vi "Wait till chilled water below.vi"(3 "Mode":T5, 5 "Traverse line In":T2 {"Carrier_2 Q (l/min)" format="%#.2f"; "Row Duration (mins)" format="%#.1f"; "Row No" min=0; "Trace Gas Concentration (%)" min=0.0 format="%#_4f"; "Carrier_1 Q (l/min)" format="%#.4f"; "Tunnel Speed" format="%#.2f"; "Start X" format="%#.2f"; "Start Y" format="%#.2f"; "Start Z" format="%#.2f"; "End X" format="%#.2f"; "End Y" format="%#.2f"; "End Z" format="%#.2f"; "Averaging time (min)" min=0.0 format="%#.2f"}) -> (0 "Error Message":string, 1 "Status":T1, 2 "Traverse line Out":T2 {"Carrier_2 Q (l/min)" format="%#.2f"; "Row Duration (mins)" format="%#.1f"; "Row No" min=0; "Trace Gas Concentration (%)" min=0.0 format="%#_4f"; "Carrier_1 Q (l/min)" format="%#.4f"; "Tunnel Speed" format="%#.2f"; "Start X" format="%#.2f"; "Start Y" format="%#.2f"; "Start Z" format="%#.2f"; "End X" format="%#.2f"; "End Y" format="%#.2f"; "End Z" format="%#.2f"; "Averaging time (min)" min=0.0 format="%#.2f"})   [LabVIEW 2020]
uses:
  Gen Trav/Multi_Run_Status.ctl
  Controls/User_Specific_mode.ctl
  ADAM Client/Sub VIs/ADAM Controls/Tunnel_speed_mode.ctl
  Gen Trav/Spacing.ctl
  Gen Trav/Traverse_cluster.ctl
  Controls/Multi_run_mode.ctl
panel:
  out "Initial Hydrosonic setting":dbl
  in  "stop":bool
  out "Chilled water temp":dbl(graph)
  out "Initial Uni Chilled water temp":dbl
  out "Initial Tunnel Speed":dbl
  # "X           Y            Z"
  # "Start"
  # "End"
  # "X           Y            Z"
  # "Start"
  # "End"
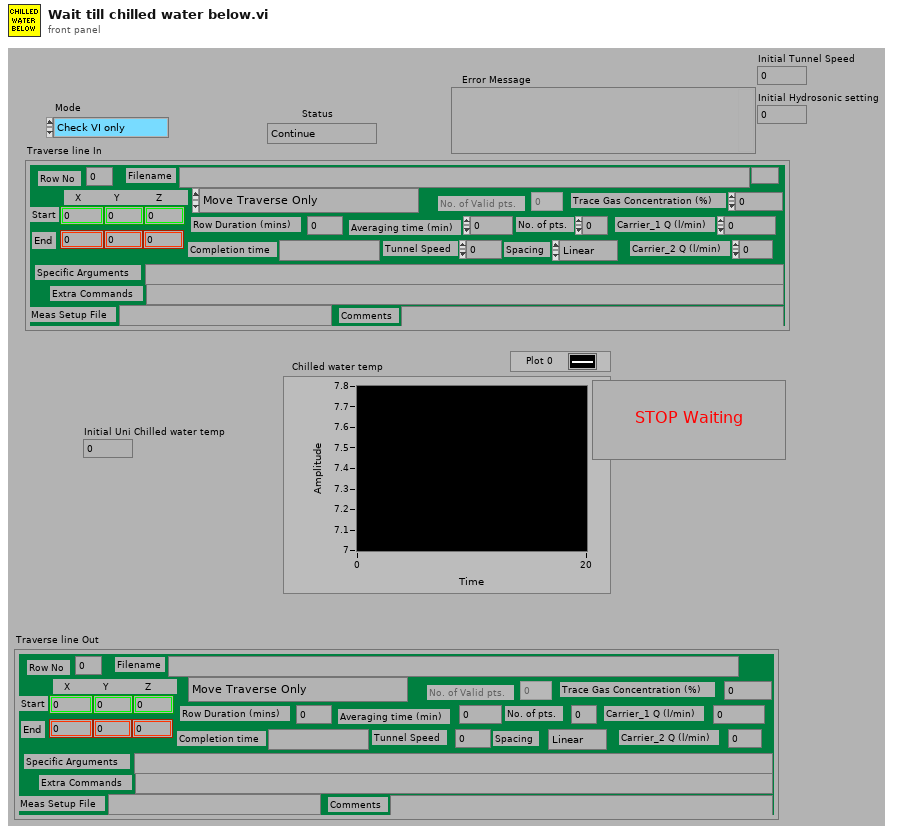
[diagram p1: front panel]
types:
  T1 = typedef "Multi_Run_Status.ctl" = enum16{"Continue", "Continue with Error", "Jump to Next Point", "Jump to Next Row", "Jump To Fall Back", "Terminate Run"}
  T2 = typedef "Traverse_cluster.ctl" = cluster{"Start X":sgl, "Start Y":sgl, "Start Z":sgl, "End X":sgl, "End Y":sgl, "End Z":sgl, "No. of pts.":i32, "Spacing":T3, "Filename":path, "Tunnel Speed":dbl, "Averaging time (min)":dbl, "Extra Commands":string, "Carrier_1 Q (l/min)":dbl, "Carrier_2 Q (l/min)":dbl, "Trace Gas Concentration (%)":dbl, "Specific Arguments":string, "Comments":string, "Row No":i32, "Row Type Selector":T4, "Completion time":string, "Row Duration (mins)":dbl, "No. of Valid pts.":i32, "Meas Setup File":string}
  T3 = typedef "Spacing.ctl" = enum16{"Linear", "Log", "Gauss", "Specified", "N/A"}
  T4 = typedef "Multi_run_mode.ctl" = enum16{"Move Traverse Only", "Set Tunnel Speed Only", "Set Source Only", "Set Measurement Conditions", "Single Measurement", "Vertical Profile", "Lateral Profile", "Longitudinal Profile", "Multi-Axis Profile", "Explore Volume", "Auto Calibrate", "Meas Fast FID Bkgnd", "Check Beam Power", "Scanning Valve Measurement", "Run VI Named:", "Set ADAM Ch", "Wait (minutes)", "Send Message", "Synchronize With:", "Fall Back to this Row", "Turn Off Row Repeating", "Traverse 3D Volume", "Blank Row", "Jump to Fall Back Row"}
  T5 = typedef "User_Specific_mode.ctl" = enum16{"Check VI only", "Run VI"}
  T6 = typedef "Tunnel_speed_mode.ctl" = enum16{"Set Speed", "Set Speed then wait", "Is tunnel speed allowable?"}
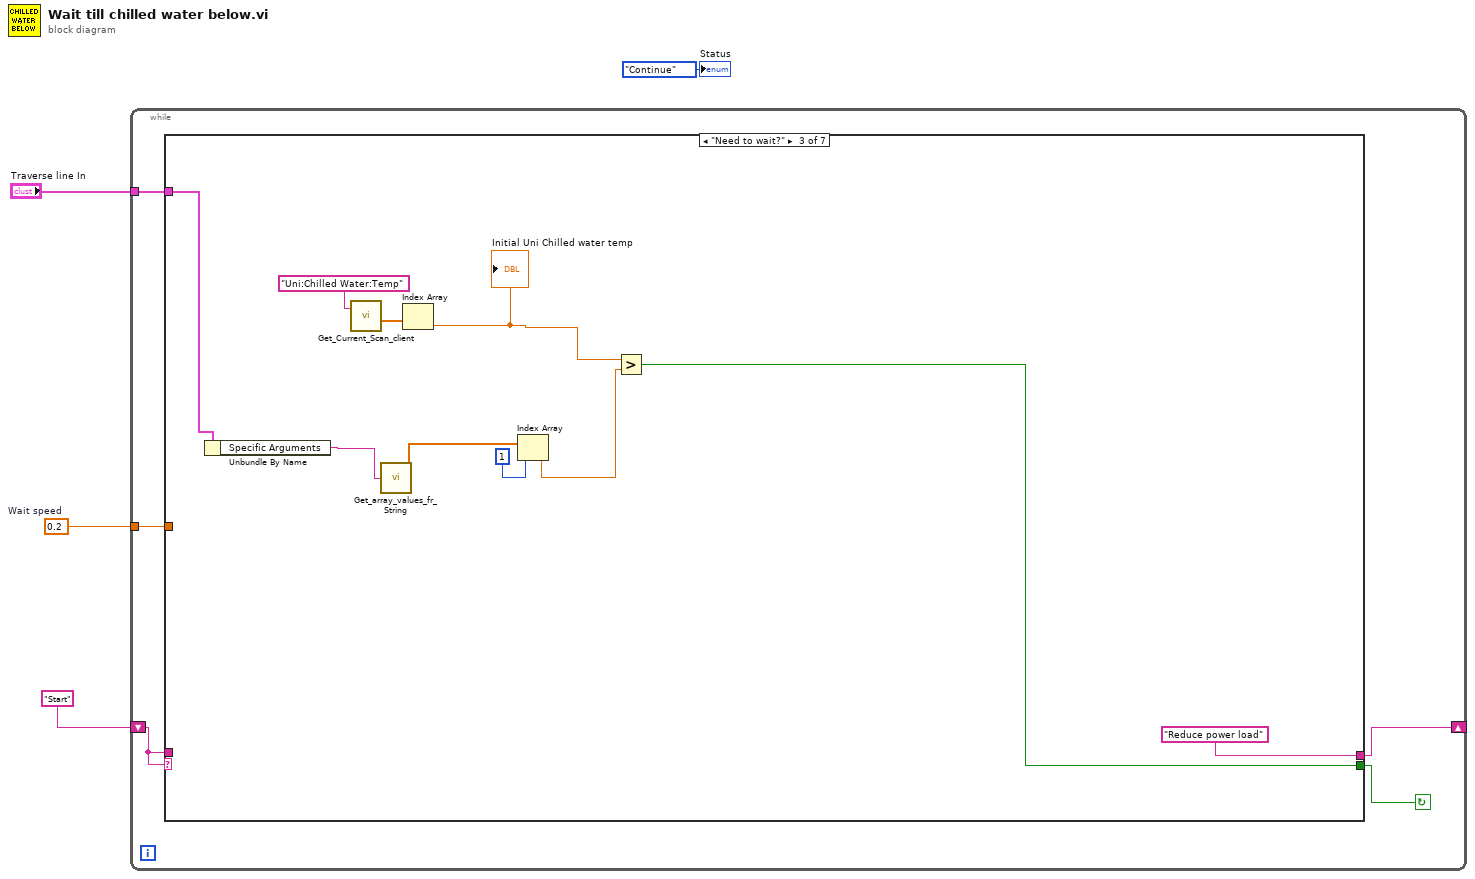
[diagram p0: block diagram]
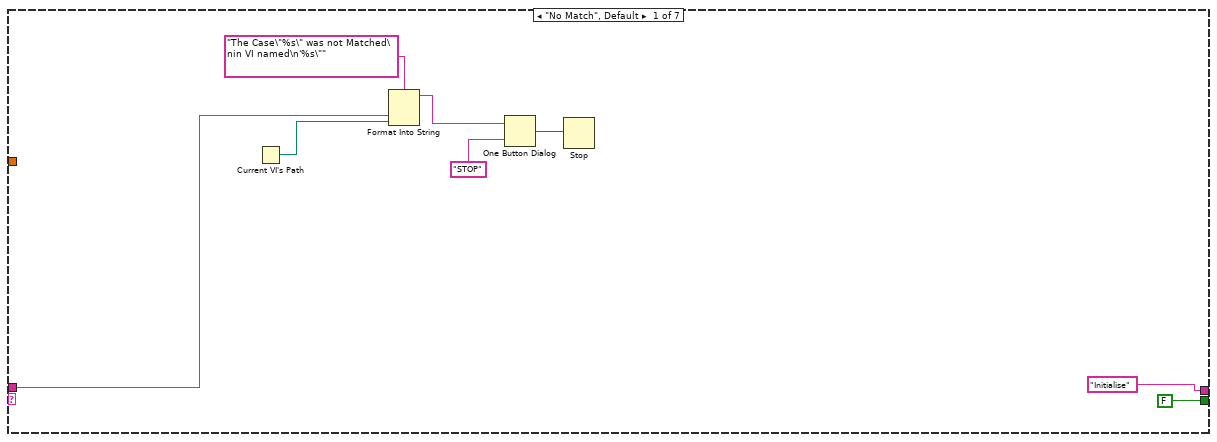
[diagram p2: hidden frame]
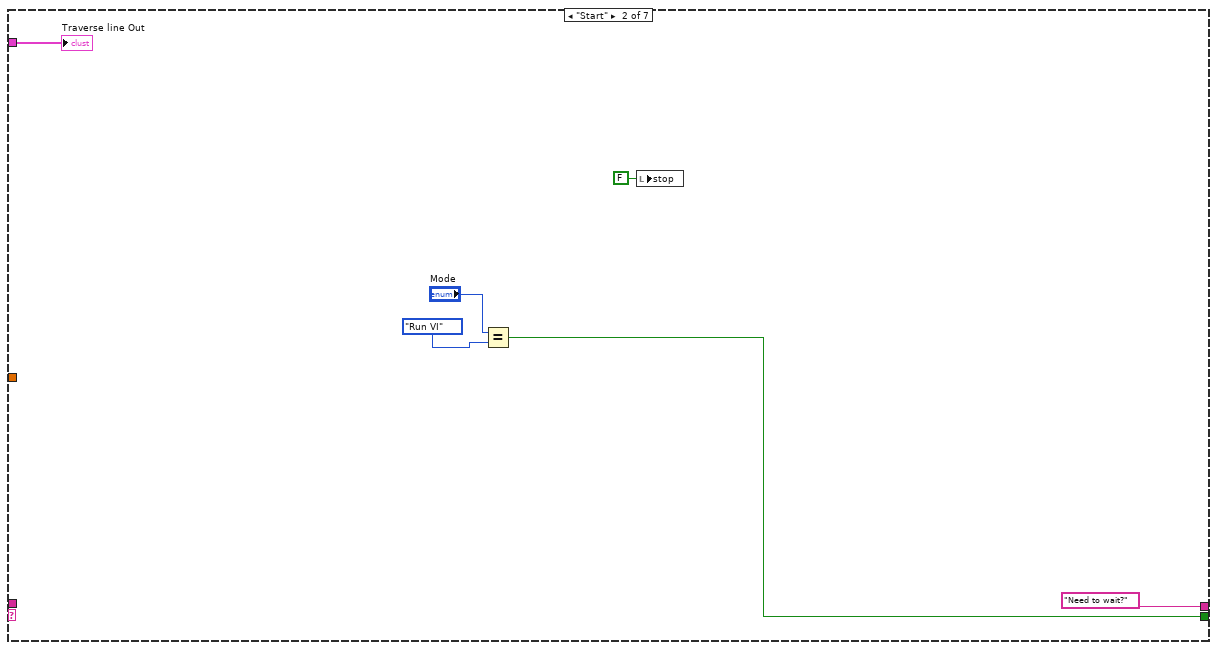
[diagram p3: hidden frame]
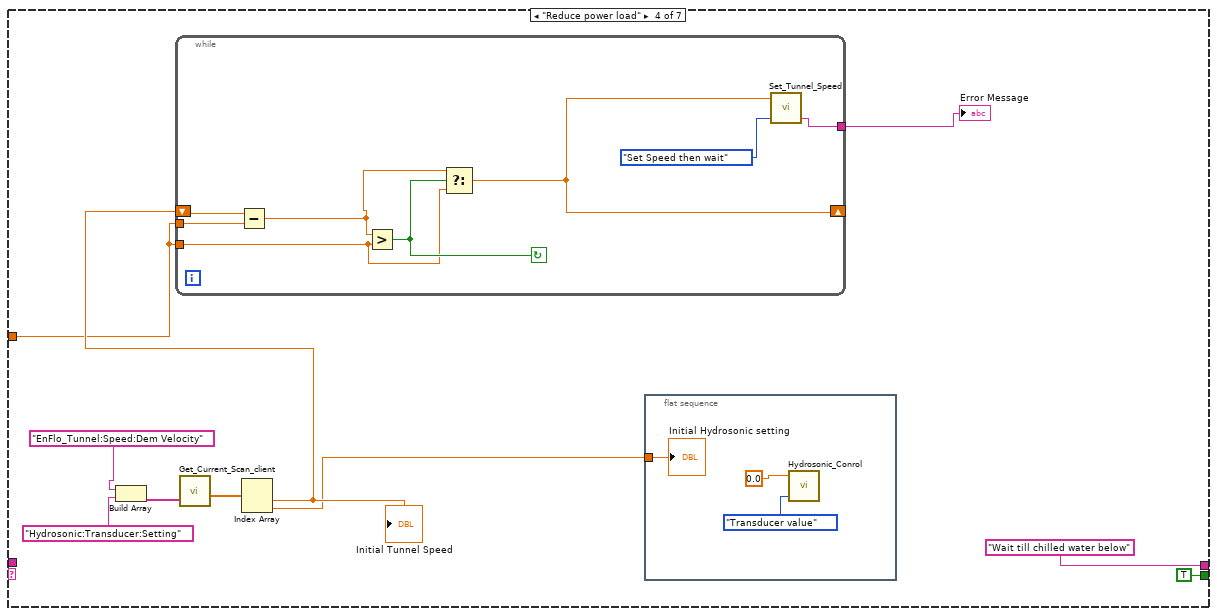
[diagram p4: hidden frame]
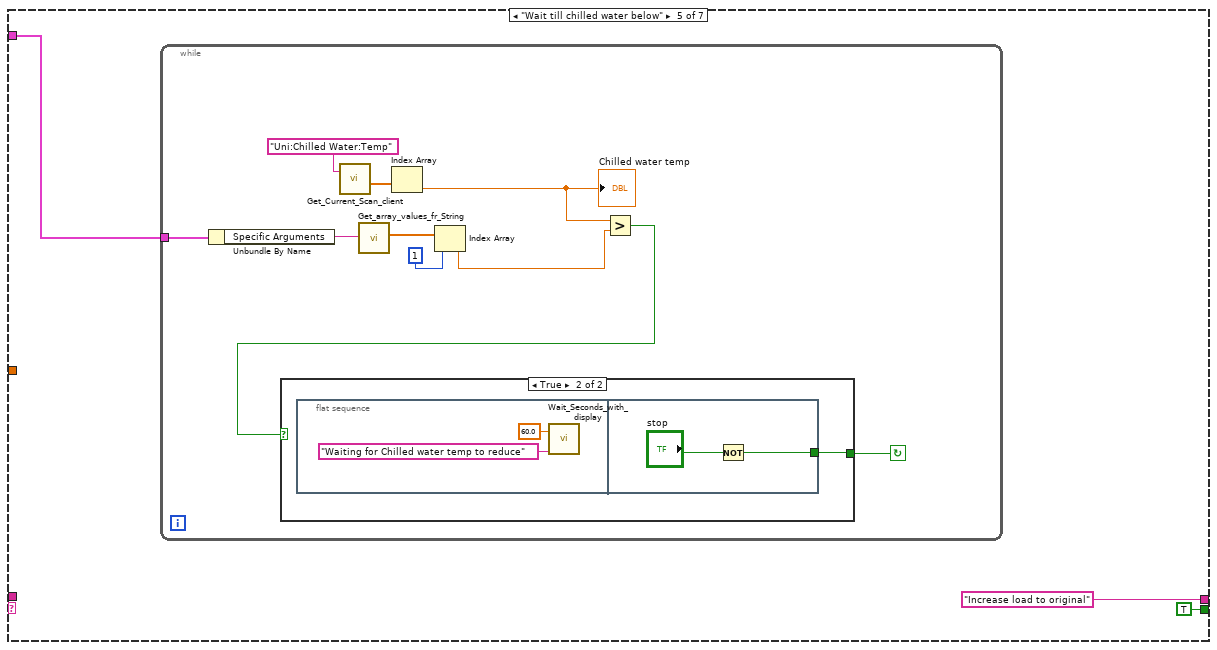
[diagram p5: hidden frame]
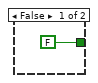
[diagram p6: hidden frame]
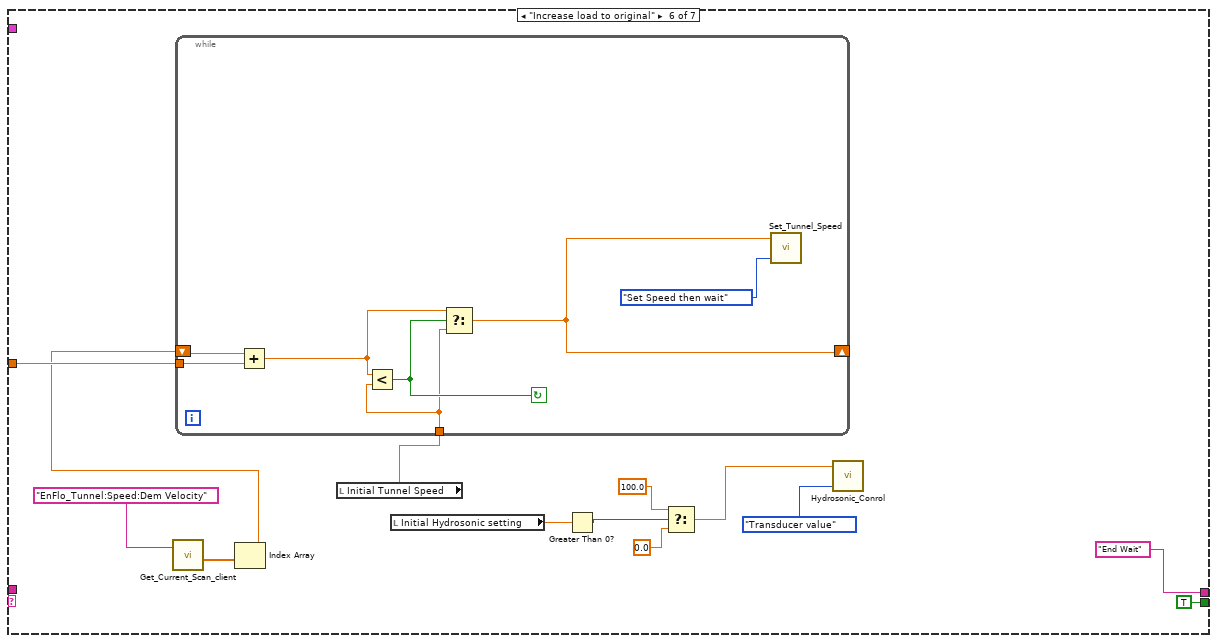
[diagram p7: hidden frame]
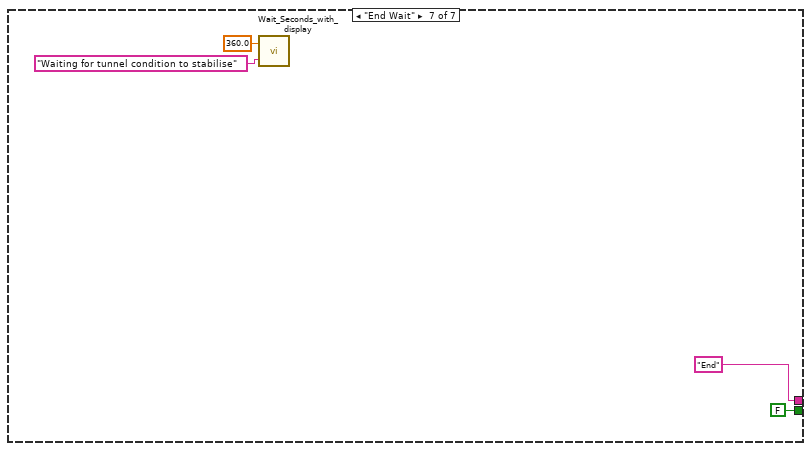
[diagram p8: hidden frame]
diagram:
  w2 = 0.2  # Wait speed
  n1 = while {
    shift-left: "Start" -> [w7]
    shift-right: [w8] -> _
    tunnel: "Traverse line In" -> [w6]
    tunnel: w2 -> [w5]
    stop <- w9 continue-if-true
    n2 = case shown="\"Need to wait?\"" w7 {
      tunnel: [FALSE w20 w26 TRUE TRUE TRUE FALSE] -> w9
      tunnel: ["Initialise" "Need to wait?" "Reduce power load" "Wait till chilled water below" "Increase load to original" "End Wait" "End"] -> w8
      tunnel: w7 -> [w12 _ _ _ _ _ _]
      tunnel: w6 -> [_ w19 w25 _ w56 _ _]
      tunnel: w5 -> [_ _ _ w38 _ w85 _]
      frame "No Match", Default {
        n3 = Current VI's Path() -> (path=w11:path)
        n4 = Format Into String(format string="The Case\"%s\" was not Matched\nin VI named\n'%s\"" ("Format String"), w12, w11) -> (resulting string=w15:string)  [unwired: 2 in, 1 out]
        n5 = One Button Dialog(message=w15, button name ("OK")="STOP") -> (true=w13:bool)
        n6 = Stop(stop? (T)=w13) -> ()
      }
      frame "Start" {
        n7 = Equal?(x="Mode", y=User_Specific_mode."Run VI" ("Mode")) -> (x = y?=w20:bool)
        n8 = local write "stop"(FALSE ("stop")) -> ()
        "Traverse line Out" <- w19
      }
      frame "Need to wait?" {
        n9 = Unbundle By Name(w25) -> ("Specific Arguments"=w30:string)
        n10 = call "Get_Current_Scan_client.vi"("singleChannel"="Uni:Chilled Water:Temp") -> ("Numerical Values"=w31:dbl[])  [unwired: 2 in, 2 out]
        n11 = call "Get_array_values_fr_String.vi"("String Value"=w30) -> ("Numeric Array"=w28:dbl[])  [unwired: 1 out]
        n12 = Index Array(array=w31) -> (element=w32:dbl)  [unwired: 1 in]
        "Initial Uni Chilled water temp" <- w32
        n13 = Index Array(array=w28, index=1) -> (element=w27:dbl)
        n14 = Greater?(x=w32, y=w27) -> (0:w26:bool)
      }
      frame "Reduce power load" {
        n15 = Build Array("EnFlo_Tunnel:Speed:Dem Velocity", "Hydrosonic:Transducer:Setting") -> (w40:string[])
        n16 = call "Get_Current_Scan_client.vi"("multipleChannels"=w40) -> ("Numerical Values"=w41:dbl[])  [unwired: 2 in, 2 out]
        n17 = Index Array(array=w41) -> (element #1=w39:dbl, element #2=w34:dbl)  [unwired: 2 in]
        "Initial Tunnel Speed" <- w39
        n18 = while {
          shift-right: [w50] -> _
          shift-left: w39 -> [w54]
          tunnel: w38 -> [w49]
          tunnel: w38 -> [w48]
          tunnel: [w47] -> w36
          stop <- w51 continue-if-true
          n19 = Subtract(x=w54, y=w49) -> (x-y=w52:dbl)
          n20 = Greater?(x=w52, y=w48) -> (0:w51:bool)
          n21 = Select(t=w52, s=w51, f=w48) -> (s? t:f=w50:dbl)
          n22 = call "Set_Tunnel_Speed.vi"("Mode"=Tunnel_speed_mode."Set Speed then wait" ("Mode 2"), "Tunnel Velocity m/s"=w50) -> ("Error String"=w47:string)  [unwired: 2 in, 1 out]
        }
        "Error Message" <- w36
        n23 = flat-sequence {
          tunnel: w34 -> [w44]
          frame #0 {
            n24 = call "Hydrosonic_Conrol.vi"("Input Mode"=enum16{"Desired Frequency", "Transducer value"}."Transducer value", "Desired Value"=0.0 ("Set output")) -> ()  [unwired: 2 in, 2 out]
            "Initial Hydrosonic setting" <- w44
          }
        }
      }
      frame "Wait till chilled water below" {
        n25 = while {
          tunnel: w56 -> [w62]
          stop <- w59 continue-if-true
          n26 = Unbundle By Name(w62) -> ("Specific Arguments"=w66:string)
          n27 = call "Get_Current_Scan_client.vi"("singleChannel"="Uni:Chilled Water:Temp") -> ("Numerical Values"=w67:dbl[])  [unwired: 2 in, 2 out]
          n28 = call "Get_array_values_fr_String.vi"("String Value"=w66) -> ("Numeric Array"=w64:dbl[])  [unwired: 1 out]
          n29 = Index Array(array=w67) -> (element=w61:dbl)  [unwired: 1 in]
          "Chilled water temp" <- w61
          n30 = Index Array(array=w64, index=1) -> (element=w63:dbl)
          n31 = Greater?(x=w61, y=w63) -> (0:w60:bool)
          n32 = case shown="True" w60 {
            tunnel: [FALSE w69] -> w59
            frame False {
            }
            frame True {
              n33 = flat-sequence {
                tunnel: [w72] -> w69
                frame #0 {
                  n34 = call "Wait_Seconds_with_display.vi"("Message"="Waiting for Chilled water temp to reduce", "Seconds to wait"=60.0) -> ()  [unwired: 1 in, 1 out]
                }
                frame #1 {
                  n35 = Not(x="stop") -> (.not. x?=w72:bool)
                }
              }
            }
          }
        }
      }
      frame "Increase load to original" {
        n36 = call "Get_Current_Scan_client.vi"("singleChannel"="EnFlo_Tunnel:Speed:Dem Velocity") -> ("Numerical Values"=w86:dbl[])  [unwired: 2 in, 2 out]
        n37 = Index Array(array=w86) -> (element=w84:dbl)  [unwired: 1 in]
        n38 = local read "Initial Tunnel Speed"() -> (w76:dbl)
        n39 = while {
          shift-right: [w89] -> _
          shift-left: w84 -> [w93]
          tunnel: w85 -> [w88]
          tunnel: w76 -> [w87]
          stop <- w90 continue-if-true
          n40 = Add(x=w93, y=w88) -> (x+y=w91:dbl)
          n41 = Less?(x=w91, y=w87) -> (x < y?=w90:bool)
          n42 = Select(t=w91, s=w90, f=w87) -> (s? t:f=w89:dbl)
          n43 = call "Set_Tunnel_Speed.vi"("Mode"=Tunnel_speed_mode."Set Speed then wait" ("Mode 2"), "Tunnel Velocity m/s"=w89) -> ()  [unwired: 2 in, 2 out]
        }
        n44 = local read "Initial Hydrosonic setting"() -> (w75:dbl)
        n45 = Greater Than 0?(x=w75) -> (x > 0?=w77:bool)
        n46 = Select(t=100.0 ("Set output"), s=w77, f=0.0 ("Set output")) -> (s? t:f=w78:dbl)
        n47 = call "Hydrosonic_Conrol.vi"("Input Mode"=enum16{"Desired Frequency", "Transducer value"}."Transducer value", "Desired Value"=w78) -> ()  [unwired: 2 in, 2 out]
      }
      frame "End Wait" {
        n48 = call "Wait_Seconds_with_display.vi"("Message"="Waiting for tunnel condition to stabilise", "Seconds to wait"=360.0) -> ()  [unwired: 1 in, 1 out]
      }
    }
  }
  "Status" <- Multi_Run_Status."Continue" ("Status")
